vi "ImageBuffInfo.vi"(8 "error in (no error)":errorcluster) -> (0 "error out":errorcluster, 1 "MRaw Bit Depth":u32, 2 "Raw Bit Depth":u32, 3 "Image Buff Info":T1, 4 "Total Frame":u32)   [LabVIEW 8.6]
doc: "Set Image Buff Info structure."
uses:
  <vilib>/Utility/error.llb/whitespace.ctl
panel:
  in  "Total Frame":u32
  in  "(M)Raw Bit Depth":enum32{"8", "10", "12", "16"}(ring)
  in  "Refer to CIH File":bool
  out "Cancel?":bool
  in  "Interleave":enum16{"MONO", "BGR", "RGB"}(ring)
  in  "Real Bit Per Pixel":u16
  in  "Byte Per Line":i32
  in  "Height":i32
  in  "Width":i32
  in  "OK":bool
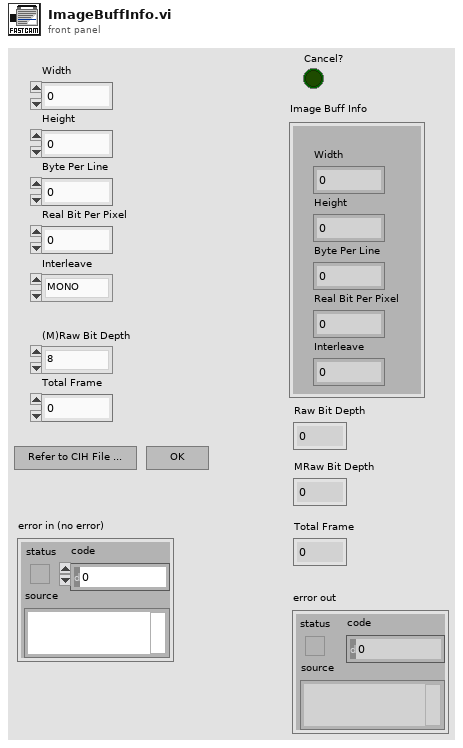
[diagram p1: front panel]
types:
  T1 = cluster{"Width":i32, "Height":i32, "Byte Per Line":i32, "Real Bit Per Pixel":u16, "Interleave":i32}
  T2 = cluster{"Width":i32, "Height":i32, "Byte Per Line":i32, "Real Bit Per Pixel":u16, i32}
  T3 = typedef "whitespace.ctl" = u16
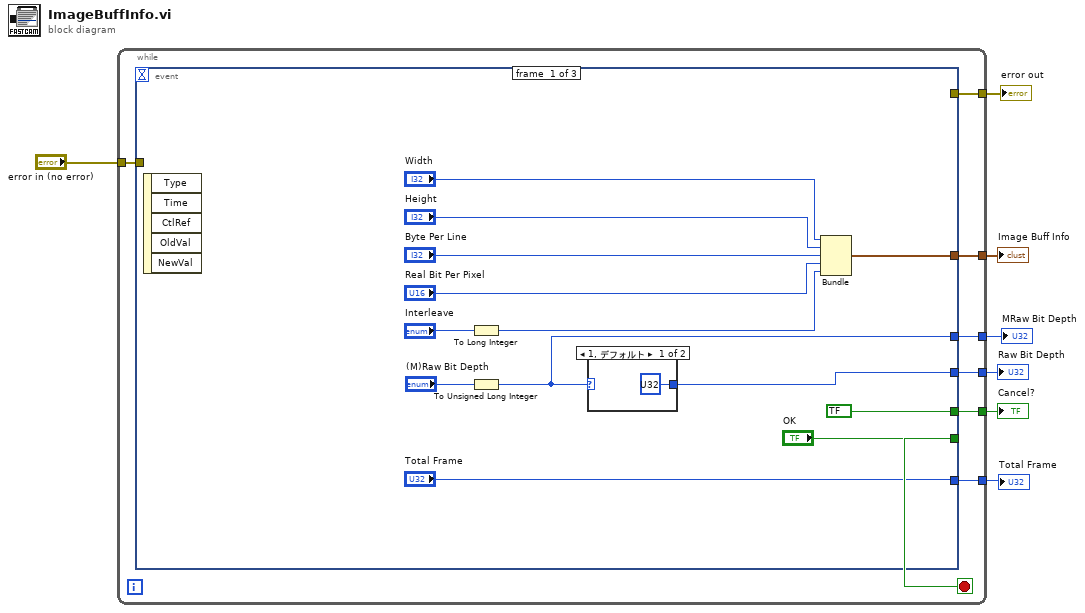
[diagram p0: block diagram]
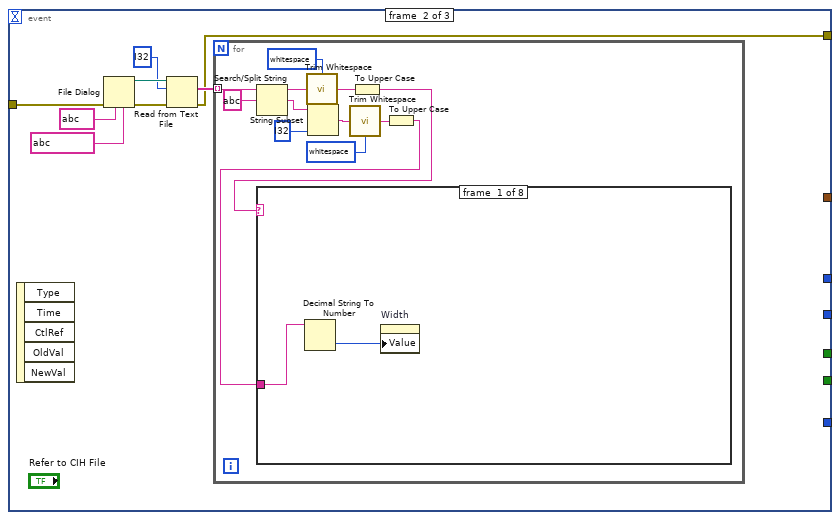
[diagram p3: hidden frame]
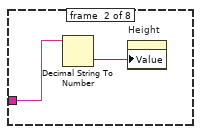
[diagram p4: hidden frame]
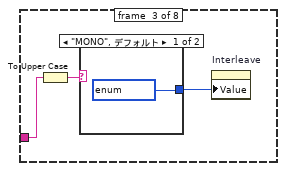
[diagram p5: hidden frame]
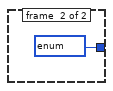
[diagram p6: hidden frame]
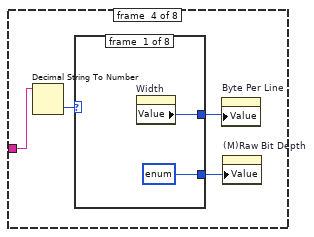
[diagram p7: hidden frame]
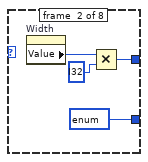
[diagram p8: hidden frame]
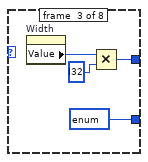
[diagram p9: hidden frame]
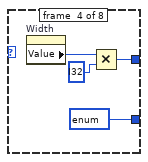
[diagram p10: hidden frame]
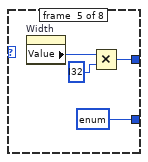
[diagram p11: hidden frame]
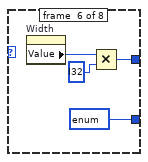
[diagram p12: hidden frame]
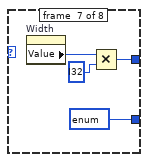
[diagram p13: hidden frame]
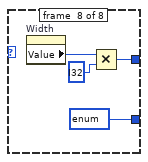
[diagram p14: hidden frame]
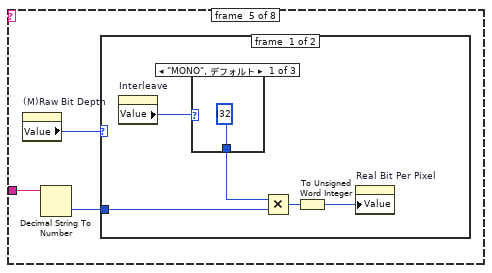
[diagram p15: hidden frame]
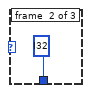
[diagram p16: hidden frame]
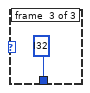
[diagram p17: hidden frame]
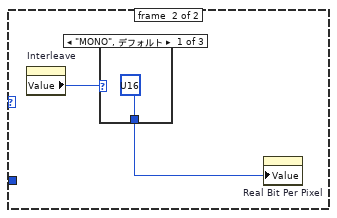
[diagram p18: hidden frame]
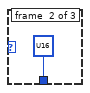
[diagram p19: hidden frame]
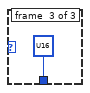
[diagram p20: hidden frame]
diagram:
  n1 = while {
    tunnel: [w15] -> w7
    tunnel: [w13] -> w6
    tunnel: [w12] -> w5
    tunnel: [w11] -> w4
    tunnel: "error in (no error)" -> [w10]
    tunnel: [w9] -> w2
    tunnel: [w8] -> w1
    stop <- w14 stop-if-true
    n2 = event shown="[1] \"Refer to CIH File\": 値変更" {
      selector: _ -> [_ _ _]
      dyn-events: _ -> [_ _ _]
      timeout: _ -> [_ _ _]
      tunnel: [bool ? _ bool ?] -> w15
      tunnel: ["OK" _ _] -> w14
      tunnel: [w22 _ _] -> w13
      tunnel: [w17 _ _] -> w12
      tunnel: [w18 _ _] -> w11
      tunnel: w10 -> [_ w32 _]
      tunnel: [_ w31 _] -> w9
      tunnel: ["Total Frame" _ _] -> w8
      event #0 {
        n3 = event-data() -> ()  [unwired: 1 in, 5 out]
        n4 = To Long Integer(number="Interleave") -> (32bit integer=w19:i32)
        n5 = To Unsigned Long Integer(number="(M)Raw Bit Depth") -> (unsigned 32bit integer=w18:u32)
        n6 = case shown="1, デフォルト" w18 {
          selector: w18 -> [_ w30]
          tunnel: [u32 ? w30] -> w17
          frame #0 {
          }
          frame #1 {
          }
        }
        n7 = Bundle("Width"="Width", "Height"="Height", "Byte Per Line"="Byte Per Line", "Real Bit Per Pixel"="Real Bit Per Pixel", w19) -> (w22:T2)  [unwired: 1 in]
      }
      event #1 {
        n8 = event-data() -> ()  [unwired: 1 in, 5 out]
        n9 = File Dialog(4:string ? ("パターンラベル"), 6:string ? ("パターン（すべてのファイル）"), 8:w32) -> (0:w35:errorcluster, 3:w36:path)  [unwired: 2 in, 4 out]
        n10 = Read from Text File(file (use dialog)=w36, count=i32 ? ("カウント"), error in=w35) -> (text=w33:string[], error out=w31:errorcluster)  [unwired: 1 in, 2 out]
        n11 = for {
          tunnel: w33 -> [w50] mode=indexing
          w45 = T3 ? items=["両方", "文字列の先頭", "文字列の終わり"] ("location (both)")
          w46 = T3 ? items=["両方", "文字列の先頭", "文字列の終わり"] ("location (both)")
          n12 = Search/Split String(string=w50, search string/char (-)=string ? ("検索文字列／文字 （-）")) -> (substring before match=w48:string, match + rest of string=w43:string)  [unwired: 1 in, 1 out]
          n13 = call <vilib>:"Trim Whitespace.vi"("string"=w48, "location (both)"=w46) -> ("trimmed string"=w47:string)
          n14 = String Subset(string=w43, offset (0)=i32 ? ("オフセット（0）")) -> (substring=w41:string)  [unwired: 1 in]
          n15 = call <vilib>:"Trim Whitespace.vi"("string"=w41, "location (both)"=w45) -> ("trimmed string"=w40:string)
          n16 = To Upper Case(1:w47) -> (0:w44:string)
          n17 = To Upper Case(1:w40) -> (0:w39:string)
          n18 = case shown="\"TOTAL FRAME\"" w44 {
            tunnel: w39 -> [w52 w54 w57 w63 w96 w112 w120 _]
            frame #0 {
              n19 = Decimal String To Number ("10進数文字列を数値に変換")(string=w52) -> (number=w51:i32)  [unwired: 2 in, 1 out]
              n20 = property on="Width" class="DigNum （指定）"("Value"=w51) -> ()  [unwired: 2 in, 2 out]
            }
            frame #1 {
              n21 = Decimal String To Number(string=w54) -> (number=w53:i32)  [unwired: 2 in, 1 out]
              n22 = property on="Height" class="DigNum （指定）"("Value"=w53) -> ()  [unwired: 2 in, 2 out]
            }
            frame #2 {
              n23 = To Upper Case(1:w57) -> (0:w56:string)
              n24 = case shown="\"MONO\", デフォルト" w56 {
                tunnel: [enum16{"MONO", "BGR", "RGB"} ? ("Interleave") enum16{"MONO", "BGR", "RGB"} ? ("Interleave")] -> w55
                frame #0 {
                }
                frame #1 {
                }
              }
              n25 = property on="Interleave" class="Enum （指定）"("Value"=w55) -> ()  [unwired: 2 in, 2 out]
            }
            frame #3 {
              n26 = Decimal String To Number(string=w63) -> (number=w62:i32)  [unwired: 2 in, 1 out]
              n27 = case shown="30" w62 {
                tunnel: [w65 w68 w72 w76 w80 w84 w88 w92] -> w61
                tunnel: [enum32{"8", "10", "12", "16"} ? ("(M)Raw Bit Depth") enum32{"8", "10", "12", "16"} ? ("(M)Raw Bit Depth") enum32{"8", "10", "12", "16"} ? ("(M)Raw Bit Depth") enum32{"8", "10", "12", "16"} ? ("(M)Raw Bit Depth") enum32{"8", "10", "12", "16"} ? ("(M)Raw Bit Depth") enum32{"8", "10", "12", "16"} ? ("(M)Raw Bit Depth") enum32{"8", "10", "12", "16"} ? ("(M)Raw Bit Depth") enum32{"8", "10", "12", "16"} ? ("(M)Raw Bit Depth")] -> w60
                frame #0 {
                  n28 = property on="Width" class="DigNum （指定）"() -> ("Value"=w65:i32)  [unwired: 2 in, 2 out]
                }
                frame #1 {
                  n29 = property on="Width" class="DigNum （指定）"() -> ("Value"=w67:i32)  [unwired: 2 in, 2 out]
                  n30 = Multiply(x=w67, y=i32 ?) -> (x*y=w68:i32)
                }
                frame #2 {
                  n31 = property on="Width" class="DigNum （指定）"() -> ("Value"=w71:i32)  [unwired: 2 in, 2 out]
                  n32 = Multiply(x=w71, y=i32 ?) -> (x*y=w72:i32)
                }
                frame #3 {
                  n33 = property on="Width" class="DigNum （指定）"() -> ("Value"=w75:i32)  [unwired: 2 in, 2 out]
                  n34 = Multiply(x=w75, y=i32 ?) -> (x*y=w76:i32)
                }
                frame #4 {
                  n35 = property on="Width" class="DigNum （指定）"() -> ("Value"=w79:i32)  [unwired: 2 in, 2 out]
                  n36 = Multiply(x=w79, y=i32 ?) -> (x*y=w80:i32)
                }
                frame #5 {
                  n37 = property on="Width" class="DigNum （指定）"() -> ("Value"=w83:i32)  [unwired: 2 in, 2 out]
                  n38 = Multiply(x=w83, y=i32 ?) -> (x*y=w84:i32)
                }
                frame #6 {
                  n39 = property on="Width" class="DigNum （指定）"() -> ("Value"=w87:i32)  [unwired: 2 in, 2 out]
                  n40 = Multiply(x=w87, y=i32 ?) -> (x*y=w88:i32)
                }
                frame #7 {
                  n41 = property on="Width" class="DigNum （指定）"() -> ("Value"=w91:i32)  [unwired: 2 in, 2 out]
                  n42 = Multiply(x=w91, y=i32 ?) -> (x*y=w92:i32)
                }
              }
              n43 = property on="Byte Per Line" class="DigNum （指定）"("Value"=w61) -> ()  [unwired: 2 in, 2 out]
              n44 = property on="(M)Raw Bit Depth" class="Enum （指定）"("Value"=w60) -> ()  [unwired: 2 in, 2 out]
            }
            frame #4 {
              n45 = property on="(M)Raw Bit Depth" class="Enum （指定）"() -> ("Value"=w95:enum32{"8", "10", "12", "16"})  [unwired: 2 in, 2 out]
              n46 = Decimal String To Number(string=w96) -> (number=w94:i32)  [unwired: 2 in, 1 out]
              n47 = case shown="\"8\"" w95 {
                tunnel: w94 -> [w97 _]
                frame #0 {
                  n48 = property on="Interleave" class="Enum （指定）"() -> ("Value"=w101:enum16{"MONO", "BGR", "RGB"})  [unwired: 2 in, 2 out]
                  n49 = case shown="\"MONO\", デフォルト" w101 {
                    tunnel: [i32 ? i32 ? i32 ?] -> w98
                    frame #0 {
                    }
                    frame #1 {
                    }
                    frame #2 {
                    }
                  }
                  n50 = Multiply(x=w98, y=w97) -> (x*y=w100:i32)
                  n51 = To Unsigned Word Integer(number=w100) -> (unsigned 16bit integer=w99:u16)
                  n52 = property on="Real Bit Per Pixel" class="DigNum （指定）"("Value"=w99) -> ()  [unwired: 2 in, 2 out]
                }
                frame #1 {
                  n53 = property on="Interleave" class="Enum （指定）"() -> ("Value"=w106:enum16{"MONO", "BGR", "RGB"})  [unwired: 2 in, 2 out]
                  n54 = case shown="\"MONO\", デフォルト" w106 {
                    tunnel: [u16 ? u16 ? u16 ?] -> w105
                    frame #0 {
                    }
                    frame #1 {
                    }
                    frame #2 {
                    }
                  }
                  n55 = property on="Real Bit Per Pixel" class="DigNum （指定）"("Value"=w105) -> ()  [unwired: 2 in, 2 out]
                }
              }
            }
            frame #5 {
              n56 = property on="(M)Raw Bit Depth" class="Enum （指定）"() -> ("Value"=w111:enum32{"8", "10", "12", "16"})  [unwired: 2 in, 2 out]
              n57 = property on="Interleave" class="Enum （指定）"() -> ("Value"=w110:enum16{"MONO", "BGR", "RGB"})  [unwired: 2 in, 2 out]
              n58 = case shown="\"LOWER\", デフォルト" w112 {
                tunnel: w111 -> [_ w114]
                tunnel: w110 -> [_ w113]
                frame #0 {
                }
                frame #1 {
                  n59 = case shown="\"10\"..\"16\", デフォルト" w114 {
                    tunnel: w113 -> [_ w116]
                    frame #0 {
                    }
                    frame #1 {
                      n60 = case shown="\"BGR\", \"RGB\"" w116 {
                        tunnel: [u16 ? u16 ?] -> w115
                        frame #0 {
                        }
                        frame #1 {
                        }
                      }
                      n61 = property on="Real Bit Per Pixel" class="DigNum （指定）"("Value"=w115) -> ()  [unwired: 2 in, 2 out]
                    }
                  }
                }
              }
            }
            frame #6 {
              n62 = Decimal String To Number ("10進数文字列を数値に変換")(string=w120) -> (offset past number=w119:i32)  [unwired: 2 in, 1 out]
              n63 = property on="Total Frame" class="DigNum （指定）"("Value"=w119) -> ()  [unwired: 2 in, 2 out]
            }
            frame #7 {
            }
          }
        }
      }
      event #2 {
        n64 = event-data() -> ()  [unwired: 1 in, 3 out]
      }
    }
  }
  "Cancel?" <- w7
  "Image Buff Info" <- w6
  "Raw Bit Depth" <- w5
  "MRaw Bit Depth" <- w4
  "error out" <- w2
  "Total Frame" <- w1
